vi "Initialize.vi"(0 "Device":string="Power Supply", 5 "Active Channel":T1, 7 "INI File Path":path, 9 "PPLs Folder Path":path, 11 "error in":errorcluster) -> (4 "Power Supply out":refnum<class "Power Supply.lvclass">, 15 "error out":errorcluster)   [LabVIEW 2018, in "Power Supply.lvlib" / "Power Supply.lvclass"]
doc: "This VI loads the power supply features from a configuration file. It typecasts the parent supply as the child class while keeping standard control of the system at the parent level. This allows developers to use parent only objects in their development which provides the abstraction layer between instrumentation and programming.\n\nInputs:\n\nDevice: (Required) Generic name of the installed device. \nActive Channel (Recommended): Only necessary for multi-channel power supplies\n\nOutputs: Typecasted power supply class"
uses:
  Power Supply.lvclass
  Custom Control/Channel List.ctl
  Power Supply.lvclass/Power Supply.ctl
  PPLs/Configuration/Configuration.lvlibp/Configuration.lvclass
  Power Supply.lvlib
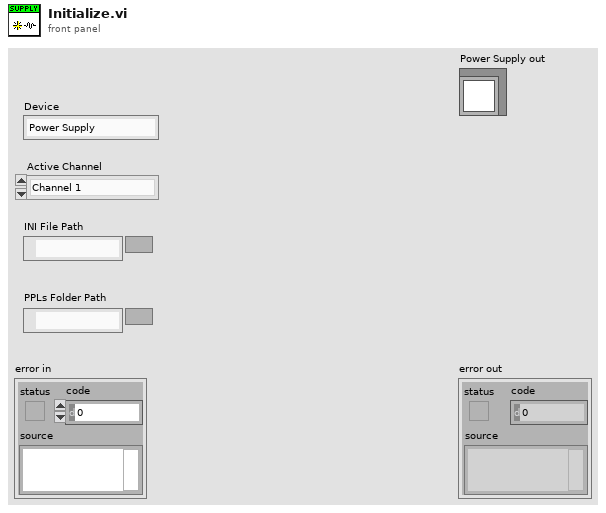
[diagram p1: front panel]
types:
  T1 = typedef "Power Supply.lvlib/Channel List.ctl" = enum16{"Channel 1", "Channel 2", "Channel 3", "Channel 4"}
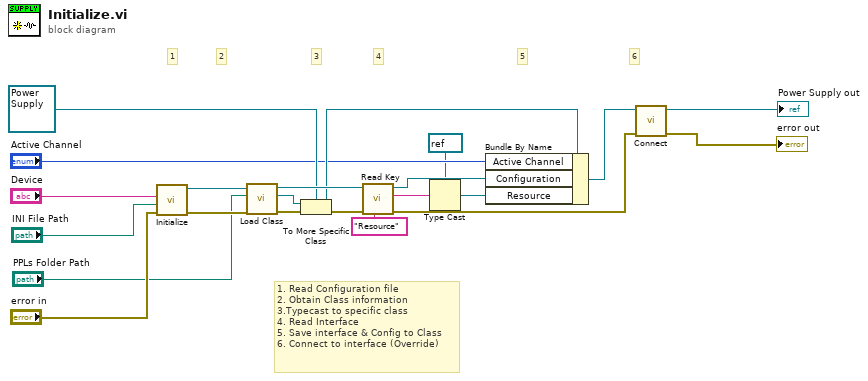
[diagram p0: block diagram]
diagram:
  # "1. Read Configuration file\n2. Obtain Class information\n3.Typecast to specific class \n4. Read Interface\n5. Save interface & Config to Class\n6. Connect to interface (Override)"
  # "6"
  # "5"
  # "4"
  # "3"
  # "2"
  # "1"
  n1 = call "Initialize.vi"("error in"="error in", "INI File Path"="INI File Path", "Device"="Device") -> ("error out"=w21:errorcluster, "Configuration out"=w19:refnum<class "Configuration.lvclass">)  [unwired: 7 in]
  n2 = call "Load Class.vi"("error in"=w21, "PPLs Folder Path"="PPLs Folder Path", "Configuration in"=w19) -> ("error out"=w12:errorcluster, "Class out"=w18:refnum<class>, "Configuration out"=w17:refnum<class "Configuration.lvclass">)  [unwired: 6 in]
  n3 = To More Specific Class(target class=refnum<class "Power Supply.lvclass"> refnum ("Power Supply in"), reference=w18, error in=w12) -> (specific class reference=w14:refnum<class "Power Supply.lvclass">, error out=w11:errorcluster)
  n4 = call "Read Key.vi"("Key:"="Resource" ("Search Value"), "error in"=w11, "Configuration in"=w17) -> ("error out"=w8:errorcluster, "Value"=w5:string, "Configuration out"=w13:refnum<class "Configuration.lvclass">)  [unwired: 6 in]
  n5 = Type Cast(type=refnum<visa-resource-name> refnum ("Resource"), x=w5) -> (*(type *) &x=w4:refnum<visa-resource-name>)
  n6 = Bundle By Name(cluster=w14, "Active Channel"="Active Channel", "Configuration"=w13, "Resource"=w4) -> (w10:refnum<class "Power Supply.lvclass">)
  n7 = call-dynamic "Connect.vi"("error in (no error)"=w8, "Power Supply in"=w10) -> ("error out"=→"error out":errorcluster, "Power Supply out"=→"Power Supply out":refnum<class "Power Supply.lvclass">)  [unwired: 8 in]
